vi "Load geometry and solve matrix.vi"(7 "STL geometry file path":path=path "C:/EnFlo Software/Anemometry/Utilities/Probe blockage potential flow sim/test stl files/Ring torus.stl", 8 "max. iters":i32=10000, 9 "res. tol.":dbl=1e-05 format="%#_6e", 10 "solver method":u8(ring)=1 items=["Jacobi (rel.)", "Jacobi (abs.)", "Gauss-Seidel (rel.)", "Gauss-Seidel (abs.)", "NI solver"], 11 "U_inf":sgl[](array[numeric])=[1.0, 0.0, 0.0]) -> (0 "Converged?":bool, 1 "Iterations":i32, 2 "sys. residual":sgl, 3 "Panel triangles out":T1[](array[typedef]), 4 "G'":sgl[](array[numeric]), 5 "N panels":i32)   [LabVIEW 2017]
uses:
  ctls/Triangle panel.ctl
  Low level/Cross product 3D_3Dpf.vi
  Low level/Unit vector_3Dpf.vi
  Low level/Dot product_3Dpf.vi
panel:
  # "26/10/17"
  # "Vertices"
  # "Edges"
  # "Unit normal"
  # "Control point"
  # "Edge\nlinks \n(tri index)"
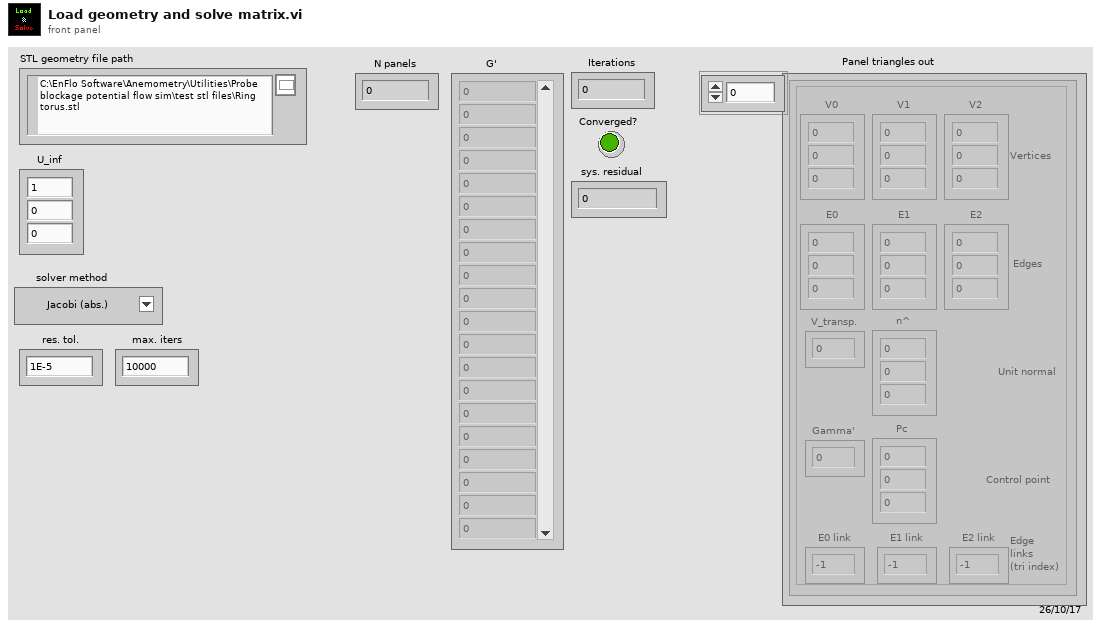
[diagram p1: front panel]
types:
  T1 = typedef "Triangle panel.ctl" = cluster{"V0":sgl[], "V1":sgl[], "V2":sgl[], "E0":sgl[], "E1":sgl[], "E2":sgl[], "n^":sgl[], "Pc":sgl[], "Gamma'":sgl, "V_transp.":sgl, "E0 link":i32, "E1 link":i32, "E2 link":i32}
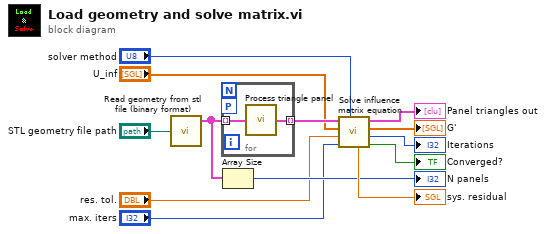
[diagram p0: block diagram]
diagram:
  n1 = call "Read geometry from stl file (binary format).vi"("STL file path"="STL geometry file path") -> ("Panel triangles array"=w11:T1[])  [unwired: 2 out]
  n2 = for {
    tunnel: w11 -> [w15] mode=indexing
    tunnel: [w14] -> w13 mode=indexing
    workers-P: _ -> [_]
    n3 = call "Process triangle panel.vi"("Panel triangle in"=w15) -> ("Panel triangle out"=w14:T1)
  }
  n4 = Array Size(array=w11) -> (size(s)=→"N panels":i32)
  n5 = call "Solve influence matrix equation.vi"("Triangle panels in"=w13, "U_inf"="U_inf", "res. tol."="res. tol.", "max. iters"="max. iters", "solver method"="solver method") -> ("sys. residual"=→"sys. residual":sgl, "Triangle panels out"=→"Panel triangles out":T1[], "G'"=→"G'":sgl[], "Iterations"=→"Iterations":i32, "Converged?"=→"Converged?":bool)  [unwired: 1 in]
